vi "Begin.vi"(8 "error in":errorcluster) -> (0 "error out":errorcluster)   [LabVIEW 2015]
doc: "Called before other user functions, this VI is expected to open initial I/O refnums, load in file data, and do all program initialization. Notice that the <B>error out</B> terminal is simply used for data flow. Wiring it to other structures or subVIs ensures that this VI runs first."
uses:
  <vilib>/Rock Robotics/WPI/DriverStation/WPI_DriverStationRobotMode2.ctl
  <vilib>/Rock Robotics/WPI/Joystick/WPI_JoystickDeviceEnum.ctl
  <vilib>/Rock Robotics/SystemInterfaces/DIO/FPGA_DIOPWMChannel.ctl
  <vilib>/Rock Robotics/SystemInterfaces/DIO/FPGA_DIOChannel.ctl
  Robot Global Data.vi
  <vilib>/Rock Robotics/Network Tables/SD Write String Array.vi
  <vilib>/Rock Robotics/WPI/MotorControl/WPI_MotorControlOpen Talon.vi
  <vilib>/Rock Robotics/WPI/Counter/WPI_CounterDigitalInputToDigitalSource.vi
  <vilib>/Rock Robotics/WPI/RobotDrive/WPI_RobotDriveOpen4MotorWithVictor.vi
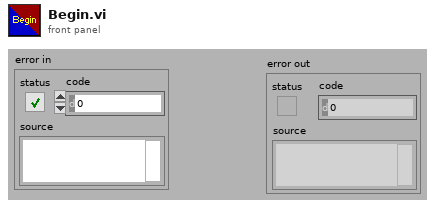
[diagram p1: front panel]
types:
  T1 = typedef "FPGA_DIOPWMChannel.ctl" = enum8{"PWM 0", "PWM 1", "PWM 2", "PWM 3", "PWM 4", "PWM 5", "PWM 6", "PWM 7", "PWM 8", "PWM 9", "PWM MXP 0", "PWM MXP 1", "PWM MXP 2", "PWM MXP 3", "PWM MXP 4", "PWM MXP 5", "PWM MXP 6", "PWM MXP 7", "PWM MXP 8", "PWM MXP 9", "Invalid"}
  T2 = typedef "FPGA_DIOChannel.ctl" = enum8{"DIO 0", "DIO 1", "DIO 2", "DIO 3", "DIO 4", "DIO 5", "DIO 6", "DIO 7", "DIO 8", "DIO 9", "DIO MXP 0", "DIO MXP 1", "DIO MXP 2", "DIO MXP 3", "DIO MXP 4", "DIO MXP 5", "DIO MXP 6", "DIO MXP 7", "DIO MXP 8", "DIO MXP 9", "DIO MXP 10", "DIO MXP 11", "DIO MXP 12", "DIO MXP 13", "DIO MXP 14", "DIO MXP 15", "Invalid"}
  T3 = typedef "WPI_JoystickDeviceEnum.ctl" = enum16{"USB 0", "USB 1", "USB 2", "USB 3", "USB 4", "USB 5"}
  T4 = typedef "WPI_DriverStationRobotMode2.ctl" = enum16{"Autonomous Disabled", "Autonomous Enabled", "Teleop Disabled", "Teleop Enabled", "Disconnected", "Finish", "Test Disabled", "Test Enabled", "Emergency Stopped"}
  T5 = typedef "WPI_DigitalInputDevRef.ctl" = cluster{"DevStatus":errorcluster, "DIO Channel":T2}
  T6 = typedef "WPI_MotorControlDeviceRef.ctl" = cluster{"DeviceStatus":errorcluster, "Type":T7, "PWM":cluster{"PWM Channel":T1, "DeadBand":T8}, "CAN":cluster{"Device Number":u8, "Control Mode":T9, "Semaphore":T10, "Max Vout":dbl, "TalonSRX Control Mode":T11}, "Invert":bool}
  T7 = typedef "WPI_MotorControlType.ctl" = enum16{"PWM", "CAN", "CANTalonSRX"}
  T8 = typedef "WPI_PWMDeadband.ctl" = cluster{"Name":string, "maxPositivePwm":i32, "minPositivePwm":i32, "centerPwm":i32, "maxNegativePwm":i32, "minNegativePwm":i32, "angularRange":u16}
  T9 = typedef "WPI_CANJaguar_ControlMode.ctl" = enum8{"Percent VBus", "Current", "Speed", "Position", "Voltage"}
  T10 = typedef "Semaphore RefNum" = refnum<k1>
  T11 = typedef "WPI_CANTalonSRX_APIControlMode.ctl" = enum8{"Percent VBus", "Speed", "Position", "Slave", "Unchanged / Invalid", "Voltage Compensation", "Current", "Motion Profile"}
  T12 = typedef "FPGA_CounterEncoderSourceConvertionLVSourceType.ctl" = cluster{"DevStatus":errorcluster, "AnalogTriggerMode?":bool, "DigitalMode":cluster{"DIO Channel":T13}, "AnalogTriggerMode":cluster{"AnalogTriggerIndex":T14, "OutputType":T15}}
  T13 = typedef "FPGA_DIODigitalSourceChannel.ctl" = enum8{"DIO 0", "DIO 1", "DIO 2", "DIO 3", "DIO 4", "DIO 5", "DIO 6", "DIO 7", "DIO 8", "DIO 9", "DIO MXP 0", "DIO MXP 1", "DIO MXP 2", "DIO MXP 3", "DIO MXP 4", "DIO MXP 5", "DIO MXP 6", "DIO MXP 7", "DIO MXP 8", "DIO MXP 9", "DIO MXP 10", "DIO MXP 11", "DIO MXP 12", "DIO MXP 13", "DIO MXP 14", "DIO MXP 15", "Disabled"}
  T14 = typedef "FPGA_AnalogTriggerIndex.ctl" = enum8{"Trig 0", "Trig 1", "Trig 2", "Trig 3", "Trig 4", "Trig 5", "Trig 6", "Trig 7", "Invalid"}
  T15 = typedef "FPGA_AnalogTriggerOutType.ctl" = enum16{"InWindow", "TriggerState", "Rising", "Falling"}
  T16 = typedef "WPI_EncoderDevRef.ctl" = cluster{"DevStatus":errorcluster, "EncoderIndex":T17, "CounterIndex":T18, "DistancePerCount":dbl, "Decoding Type":T19}
  T17 = typedef "FPGA_EncoderIdx.ctl" = enum8{"Enc 0", "Enc 1", "Enc 2", "Enc 3", "Enc 4", "Enc 5", "Enc 6", "Enc 7", "Invalid"}
  T18 = typedef "FPGA_CounterCtrSystemIndex.ctl" = enum8{"Ctr 0", "Ctr 1", "Ctr 2", "Ctr 3", "Ctr 4", "Ctr 5", "Ctr 6", "Ctr 7", "Invalid"}
  T19 = typedef "WPI_EncoderType.ctl" = enum16{"1x", "2x", "4x"}
  T20 = typedef "WPI_JoystickDevRef.ctl" = cluster{"Device":T3}
  T21 = typedef "WPI_RobotDriveDevRef.ctl" = cluster{"DevStatus":errorcluster, "Motors[]":T6[], "Square Inputs":bool, "Max Output":dbl}
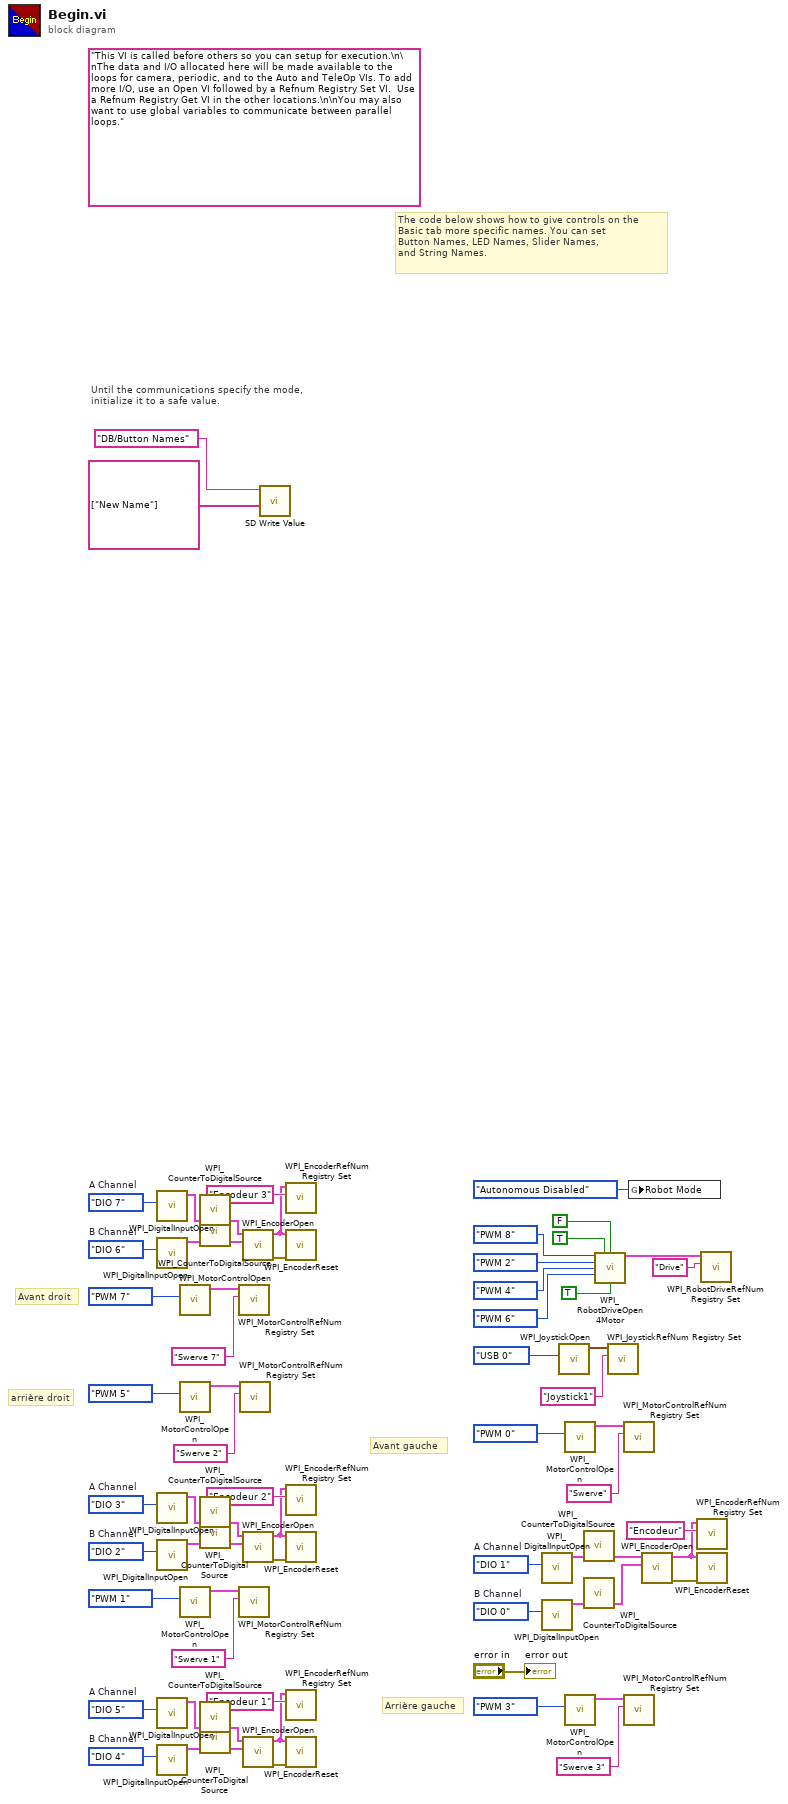
[diagram p0: block diagram]
diagram:
  w21 = FPGA_DIOChannel."DIO 6"  # B Channel
  w20 = FPGA_DIOChannel."DIO 7"  # A Channel
  w31 = FPGA_DIOChannel."DIO 2"  # B Channel
  w30 = FPGA_DIOChannel."DIO 3"  # A Channel
  w41 = FPGA_DIOChannel."DIO 4"  # B Channel
  w40 = FPGA_DIOChannel."DIO 5"  # A Channel
  w57 = FPGA_DIOChannel."DIO 0"  # B Channel
  w56 = FPGA_DIOChannel."DIO 1"  # A Channel
  (unwired) "This VI is called before others so you can setup for execution.\n\nThe data and I/O allocated here will be made available to the loops for camera, periodic, and to the Auto and TeleOp VIs. To add more I/O, use an Open VI followed by a Refnum Registry Set VI.  Use a Refnum Registry Get VI in the other locations.\n\nYou may also want to use global variables to communicate between parallel loops."
  # "Avant gauche"
  # "Arrière gauche"
  # "arrière droit"
  # "Avant droit"
  # "The code below shows how to give controls on the\nBasic tab more specific names. You can set\nButton Names, LED Names, Slider Names,\nand String Names."
  # "Until the communications specify the mode,\ninitialize it to a safe value."
  n1 = call <vilib>:"WPI_DigitalInputOpen.vi"("DIO Channel"=w20) -> ("DigitalInputDevRef"=w17:T5)  [unwired: 1 in, 9 out]
  n2 = call <vilib>:"WPI_DigitalInputOpen.vi"("DIO Channel"=w21) -> ("DigitalInputDevRef"=w18:T5)  [unwired: 1 in, 9 out]
  n3 = call <vilib>:"WPI_DigitalInputOpen.vi"("DIO Channel"=w30) -> ("DigitalInputDevRef"=w27:T5)  [unwired: 1 in, 9 out]
  n4 = call <vilib>:"WPI_DigitalInputOpen.vi"("DIO Channel"=w31) -> ("DigitalInputDevRef"=w28:T5)  [unwired: 1 in, 9 out]
  n5 = call <vilib>:"WPI_DigitalInputOpen.vi"("DIO Channel"=w40) -> ("DigitalInputDevRef"=w37:T5)  [unwired: 1 in, 9 out]
  n6 = call <vilib>:"WPI_DigitalInputOpen.vi"("DIO Channel"=w41) -> ("DigitalInputDevRef"=w38:T5)  [unwired: 1 in, 9 out]
  n7 = call-poly <vilib>:"WPI_MotorControlOpen.vi"("PWM Channel"=FPGA_DIOPWMChannel."PWM 7") -> ("MotorControlDeviceRef"=w14:T6)  [unwired: 9 in, 1 out]
  n8 = call-poly <vilib>:"WPI_MotorControlOpen.vi"("PWM Channel"=FPGA_DIOPWMChannel."PWM 5") -> ("MotorControlDeviceRef"=w33:T6)  [unwired: 9 in, 1 out]
  n9 = call-poly <vilib>:"WPI_MotorControlOpen.vi"("PWM Channel"=FPGA_DIOPWMChannel."PWM 1") -> ("MotorControlDeviceRef"=w43:T6)  [unwired: 9 in, 1 out]
  n10 = call-poly <vilib>:"WPI_CounterToDigitalSource.vi"("DigitalInputDevRef"=w17) -> ("Digital Source"=w16:T12)  [unwired: 6 out]
  n11 = call-poly <vilib>:"WPI_CounterToDigitalSource.vi"("DigitalInputDevRef"=w18) -> ("Digital Source"=w19:T12)  [unwired: 6 out]
  n12 = call-poly <vilib>:"WPI_CounterToDigitalSource.vi"("DigitalInputDevRef"=w27) -> ("Digital Source"=w26:T12)  [unwired: 6 out]
  n13 = call-poly <vilib>:"WPI_CounterToDigitalSource.vi"("DigitalInputDevRef"=w28) -> ("Digital Source"=w29:T12)  [unwired: 6 out]
  n14 = call-poly <vilib>:"WPI_CounterToDigitalSource.vi"("DigitalInputDevRef"=w37) -> ("Digital Source"=w36:T12)  [unwired: 6 out]
  n15 = call-poly <vilib>:"WPI_CounterToDigitalSource.vi"("DigitalInputDevRef"=w38) -> ("Digital Source"=w39:T12)  [unwired: 6 out]
  n16 = call <vilib>:"WPI_MotorControlRefNum Registry Set.vi"("refnum name"="Swerve 7", "MotorControlDevRef"=w14) -> ()  [unwired: 8 in, 2 out]
  n17 = call <vilib>:"WPI_MotorControlRefNum Registry Set.vi"("refnum name"="Swerve 1", "MotorControlDevRef"=w43) -> ()  [unwired: 8 in, 2 out]
  n18 = call <vilib>:"WPI_MotorControlRefNum Registry Set.vi"("refnum name"="Swerve 2", "MotorControlDevRef"=w33) -> ()  [unwired: 8 in, 2 out]
  n19 = call <vilib>:"WPI_EncoderOpen.vi"("BSource"=w19, "ASource"=w16) -> ("error out"=w9:errorcluster, "EncoderDevRef"=w8:T16)  [unwired: 6 in, 2 out]
  n20 = call <vilib>:"WPI_EncoderOpen.vi"("BSource"=w29, "ASource"=w26) -> ("error out"=w5:errorcluster, "EncoderDevRef"=w4:T16)  [unwired: 6 in, 2 out]
  n21 = call <vilib>:"WPI_EncoderOpen.vi"("BSource"=w39, "ASource"=w36) -> ("error out"=w7:errorcluster, "EncoderDevRef"=w6:T16)  [unwired: 6 in, 2 out]
  n22 = call-poly <vilib>:"SD Write Value.vi"("String Array"=string[] ["New Name"], "Name"="DB/Button Names") -> ()  [unwired: 8 in, 2 out]
  n23 = call <vilib>:"WPI_EncoderRefNum Registry Set.vi"("refnum name"="Encodeur 3", "EncoderDevRef"=w8) -> ()  [unwired: 8 in, 2 out]
  n24 = call <vilib>:"WPI_EncoderReset.vi"("error in (no error)"=w9, "EncoderDevRef"=w8) -> ()  [unwired: 8 in, 2 out]
  n25 = call <vilib>:"WPI_EncoderRefNum Registry Set.vi"("refnum name"="Encodeur 2", "EncoderDevRef"=w4) -> ()  [unwired: 8 in, 2 out]
  n26 = call <vilib>:"WPI_EncoderReset.vi"("error in (no error)"=w5, "EncoderDevRef"=w4) -> ()  [unwired: 8 in, 2 out]
  n27 = call <vilib>:"WPI_EncoderRefNum Registry Set.vi"("refnum name"="Encodeur 1", "EncoderDevRef"=w6) -> ()  [unwired: 8 in, 2 out]
  n28 = call <vilib>:"WPI_EncoderReset.vi"("error in (no error)"=w7, "EncoderDevRef"=w6) -> ()  [unwired: 8 in, 2 out]
  n29 = call <vilib>:"WPI_DigitalInputOpen.vi"("DIO Channel"=w56) -> ("DigitalInputDevRef"=w53:T5)  [unwired: 1 in, 9 out]
  n30 = call <vilib>:"WPI_DigitalInputOpen.vi"("DIO Channel"=w57) -> ("DigitalInputDevRef"=w54:T5)  [unwired: 1 in, 9 out]
  n31 = call <vilib>:"WPI_JoystickOpen.vi"("JoystickDevice"=WPI_JoystickDeviceEnum."USB 0") -> ("JoystickDevRef"=w63:T20)  [unwired: 10 in]
  n32 = call-poly <vilib>:"WPI_MotorControlOpen.vi"("PWM Channel"=FPGA_DIOPWMChannel."PWM 0") -> ("MotorControlDeviceRef"=w59:T6)  [unwired: 9 in, 1 out]
  n33 = call-poly <vilib>:"WPI_MotorControlOpen.vi"("PWM Channel"=FPGA_DIOPWMChannel."PWM 3") -> ("MotorControlDeviceRef"=w23:T6)  [unwired: 9 in, 1 out]
  n34 = call-poly <vilib>:"WPI_CounterToDigitalSource.vi"("DigitalInputDevRef"=w53) -> ("Digital Source"=w52:T12)  [unwired: 6 out]
  n35 = call-poly <vilib>:"WPI_CounterToDigitalSource.vi"("DigitalInputDevRef"=w54) -> ("Digital Source"=w55:T12)  [unwired: 6 out]
  n36 = call-poly <vilib>:"WPI_RobotDriveOpen4Motor.vi"("Rear Left Motor"=FPGA_DIOPWMChannel."PWM 8", "Rear Left Motor Inverted"=TRUE, "Rear Right Motor Inverted"=FALSE, "Rear Right Motor"=FPGA_DIOPWMChannel."PWM 2", "Front Left Motor"=FPGA_DIOPWMChannel."PWM 4", "Front Right Motor"=FPGA_DIOPWMChannel."PWM 6", "Front Right Motor Inverted"=TRUE) -> ("RobotDriveDevRef"=w46:T21)  [unwired: 7 in, 1 out]
  n37 = call <vilib>:"WPI_JoystickRefNum Registry Set.vi"("refnum name"="Joystick1", "JoystickDevRef"=w63) -> ()  [unwired: 8 in, 2 out]
  n38 = call <vilib>:"WPI_MotorControlRefNum Registry Set.vi"("refnum name"="Swerve", "MotorControlDevRef"=w59) -> ()  [unwired: 8 in, 2 out]
  n39 = call <vilib>:"WPI_MotorControlRefNum Registry Set.vi"("refnum name"="Swerve 3", "MotorControlDevRef"=w23) -> ()  [unwired: 8 in, 2 out]
  n40 = global write "Robot Global Data.vi" "Robot Mode"(WPI_DriverStationRobotMode2."Autonomous Disabled" ("Robot Mode")) -> ()
  n41 = call <vilib>:"WPI_EncoderOpen.vi"("BSource"=w55, "ASource"=w52) -> ("error out"=w11:errorcluster, "EncoderDevRef"=w10:T16)  [unwired: 6 in, 2 out]
  n42 = call <vilib>:"WPI_EncoderRefNum Registry Set.vi"("refnum name"="Encodeur", "EncoderDevRef"=w10) -> ()  [unwired: 8 in, 2 out]
  n43 = call <vilib>:"WPI_EncoderReset.vi"("error in (no error)"=w11, "EncoderDevRef"=w10) -> ()  [unwired: 8 in, 2 out]
  n44 = call <vilib>:"WPI_RobotDriveRefNum Registry Set.vi"("refnum name"="Drive", "RobotDriveDevRef"=w46) -> ()  [unwired: 8 in, 2 out]
  "error out" <- "error in"
